vi "Save Ctl Image to File.vi"(8 "error in":errorcluster, 11 "LabVIEW File with Button":path) -> (0 "error out":errorcluster, 3 "File with Button (dup)":path)   [LabVIEW 2021]
doc: "This example VI was obtained from this post: \n\nhttps://forums.ni.com/t5/LabVIEW-APIs-Discussions/Set-TRUE-FALSE-Image-of-a-boolean-control-automatically-using/m-p/3419083/highlight/true#M868\n\n<b>WARNING</b>\nThis VI uses a dll call to the resource file for a LabVIEW VI/CTL - it is searching the binary data for the PNG images that the VI or CTL contains\n\n<b>Code Developed By:</b> +\nDaniel Coons +\nTechnology Service Corporation +\nwww.tsc.com/atcs"
panel:
  out "Array":string[](array[string])
  in  "Save dir":path
  out "Resources":string[](array[string])
  # "For DEBUG"
  # "MNGI resources are 6 images\non buttons (pressed, hover, etc)"
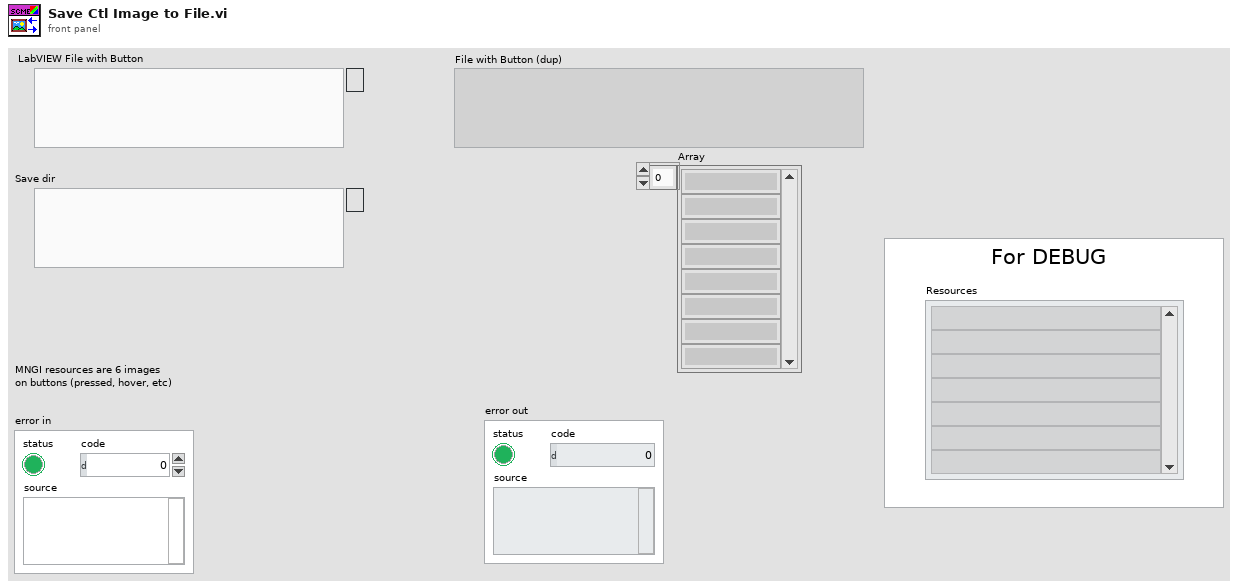
[diagram p1: front panel]
types:
  T1 = cluster{"type":u32, "id":i32, "name":string, "binary data":string}[]
  T2 = enum16{"open", "replace", "create", "open or create", "replace or create", "replace or create with confirmation"}
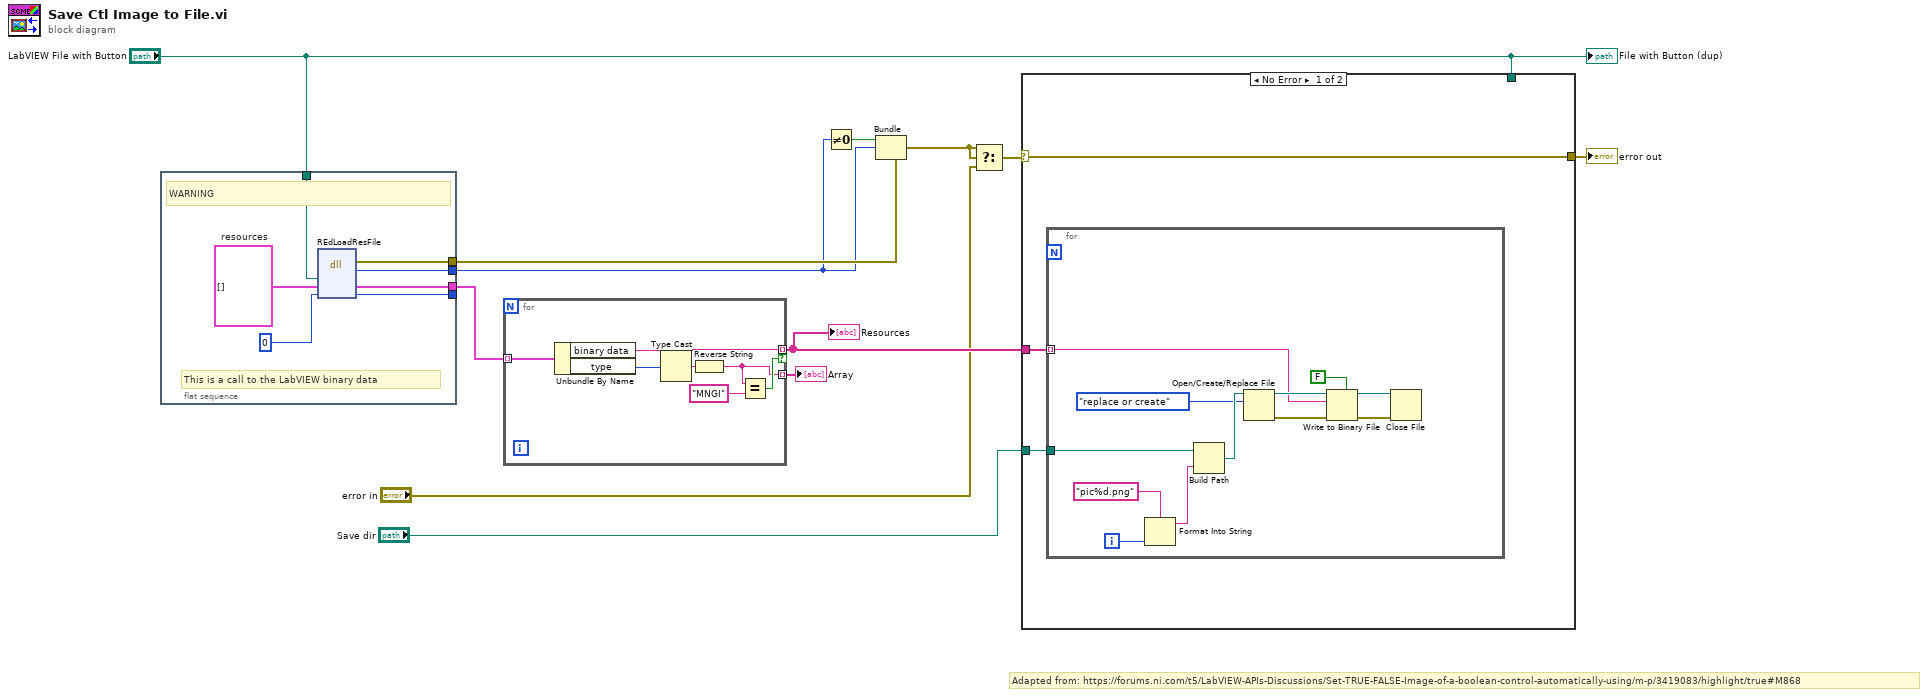
[diagram p0: block diagram]
diagram:
  # "Adapted from: https://forums.ni.com/t5/LabVIEW-APIs-Discussions/Set-TRUE-FALSE-Image-of-a-boolean-control-automatically-using/m-p/3419083/highlight/true#M868"
  n1 = flat-sequence {
    tunnel: [w17] -> w12
    tunnel: [w16] -> w10
    tunnel: [w15] -> _
    tunnel: [w14] -> w9
    tunnel: "LabVIEW File with Button" -> [w13]
    frame #0 {
      w19 = T1 []  # resources
      # "This is a call to the LabVIEW binary data"
      # "WARNING"
      n2 = dll-call lib="LabVIEW" fn="REdLoadResFile"("path"=w13, "resources"=w19, "type"=0) -> (error out=w17:errorcluster, "return type"=w16:i32, "resources"=w14:T1, "type"=w15:i32)  [unwired: 3 in, 2 out]
    }
  }
  n3 = for {
    tunnel: w9 -> [w26] mode=indexing
    tunnel: [w21] -> w5 mode=indexing if=w23
    tunnel: [w20] -> w1 mode=indexing
    n4 = Unbundle By Name(w26) -> ("binary data"=w21:string, "type"=w24:u32)
    n5 = Type Cast(x=w24) -> (*(type *) &x=w25:string)  [unwired: 1 out]
    n6 = Reverse String(1:w25) -> (0:w20:string)
    n7 = Equal?(x=w20, y="MNGI") -> (x = y?=w23:bool)
  }
  "Resources" <- w5
  "Array" <- w1
  n8 = Not Equal To 0?(x=w10) -> (x != 0?=w11:bool)
  n9 = Bundle(cluster=w12, "status"=w11, "code"=w10) -> (w8:errorcluster)  [unwired: 1 out]
  n10 = Select(t=w8, s=w8, f="error in") -> (s? t:f=w7:errorcluster)
  n11 = case shown="No Error" w7 {
    selector: w7 -> [w29 w42]
    tunnel: [w29 w42] -> w3
    tunnel: "LabVIEW File with Button" -> [_ _]
    tunnel: w5 -> [w28 _]
    tunnel: "Save dir" -> [w27 _]
    frame No Error {
      n12 = for {
        tunnel: w28 -> [w36] mode=indexing
        tunnel: w27 -> [w32]
        i -> [w35]
        n13 = Format Into String(format string="pic%d.png", w35) -> (resulting string=w33:string)  [unwired: 2 in, 1 out]
        n14 = Build Path(base path=w32, name or relative path=w33) -> (appended path=w31:path)
        n15 = Open/Create/Replace File(file path (use dialog)=w31, operation (0:open)=T2."replace or create") -> (refnum out=w37:refnum<file>, error out=w38:errorcluster)  [unwired: 4 in, 1 out]
        n16 = Write to Binary File(file (use dialog)=w37, data=w36, error in=w38, 5:FALSE ("prepend array or string size? (T)")) -> (refnum out=w39:refnum<file>, error out=w40:errorcluster)  [unwired: 2 in, 1 out]
        n17 = Close File(refnum=w39, error in=w40) -> ()  [unwired: 2 out]
      }
    }
    frame Error {
    }
  }
  "error out" <- w3
  "File with Button (dup)" <- "LabVIEW File with Button"
